vi "Read Gesture.vi"(8 "error in (no error)":errorcluster, 11 "Gesture Sensor in":refnum<class "Gesture Sensor.lvclass">) -> (0 "error out":errorcluster, 2 "Gesture":T1, 3 "Gesture Sensor out":refnum<class "Gesture Sensor.lvclass">)   [LabVIEW 2020, in "CTI-Peripheral.lvlib" / "Gesture Sensor.lvclass"]
uses:
  Gesture Sensor.lvclass
  Gesture.ctl
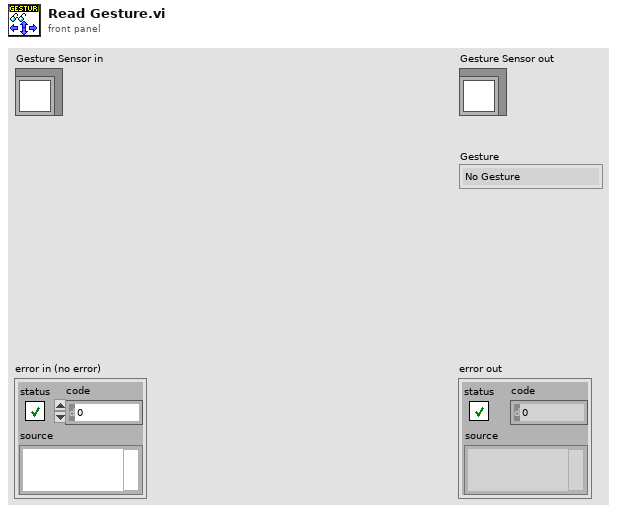
[diagram p1: front panel]
types:
  T1 = typedef "CTI-Peripheral.lvlib/Gesture Sensor.lvclass/Gesture.ctl" = enum16{"No Gesture", "Up", "Down", "Left", "Right", "Forward", "Backward", "Clockwise", "Counterclockwise"}
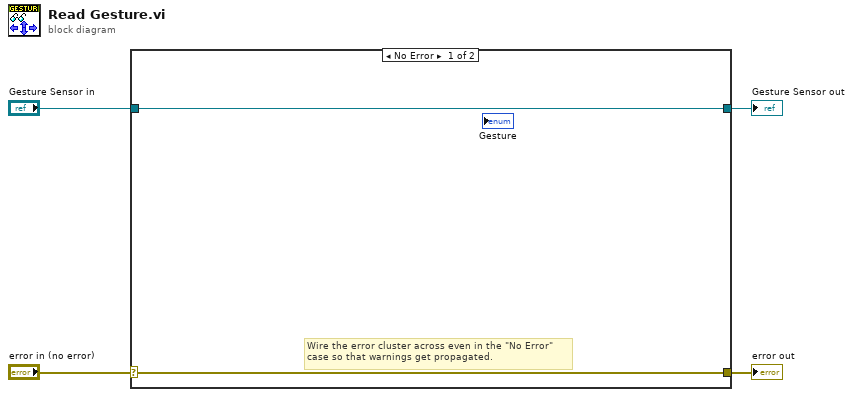
[diagram p0: block diagram]
diagram:
  n1 = case shown="No Error" "error in (no error)" {
    selector: "error in (no error)" -> [w5 w8]
    tunnel: [w5 w8] -> w3
    tunnel: [w6 w7] -> w1
    tunnel: "Gesture Sensor in" -> [w6 w7]
    frame No Error {
      # "Wire the error cluster across even in the \"No Error\"\ncase so that warnings get propagated."
    }
    frame Error {
    }
  }
  "error out" <- w3
  "Gesture Sensor out" <- w1
